vi "API - Initialize Connection to DAQ.vi"(8 "error in":errorcluster, 11 "DAQ IP Address":string="192.168.1.1") -> (0 "error out":errorcluster, 3 "TCP Network Connection out":refnum<k5>)   [LabVIEW 2020]
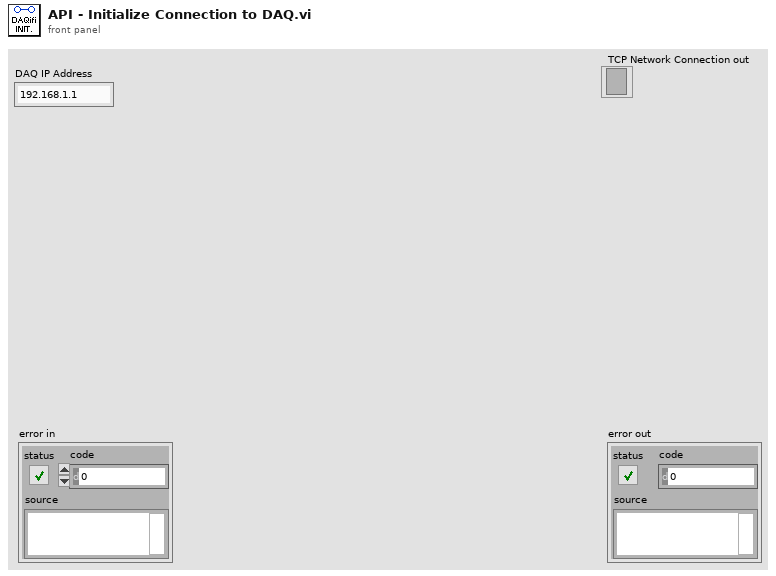
[diagram p1: front panel]
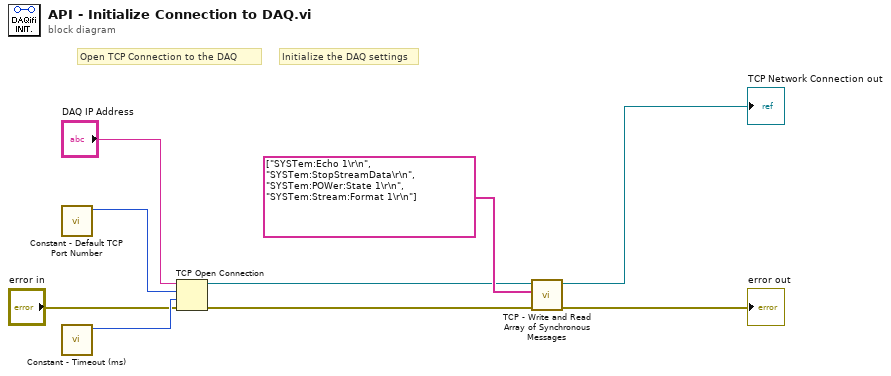
[diagram p0: block diagram]
diagram:
  # "Open TCP Connection to the DAQ"
  # "Initialize the DAQ settings"
  n1 = call "Constant - Default TCP Port Number.vi"() -> ("Port"=w8:u16)  [unwired: 11 in]
  n2 = call "Constant - Timeout (ms).vi"() -> ("timeout (ms)"=w4:i32)  [unwired: 11 in]
  n3 = TCP Open Connection(address="DAQ IP Address", remote port or service name=w8, timeout ms (60000)=w4, error in (no error)="error in") -> (connection ID=w5:refnum<k5>, error out=w6:errorcluster)  [unwired: 1 in]
  n4 = call "TCP - Write and Read Array of Synchronous Messages.vi"("error in"=w6, "Array of Messages to Send"=string[] ["SYSTem:Echo 1\r\n", "SYSTem:StopStreamData\r\n", "SYSTem:POWer:State 1\r\n", "SYSTem:Stream:Format 1\r\n"], "TCP Network Connection in"=w5) -> ("error out"=→"error out":errorcluster, "TCP Network Connection out"=→"TCP Network Connection out":refnum<k5>)  [unwired: 6 in, 1 out]
